vi "Sequence.BuildPreviewWaveform.vi"(7 "WaveformGraph in":refnum<vi>, 8 "error in (no error)":errorcluster, 9 "Rows":cluster{"Start Index":i32, "Length":i32}={"Start Index"=0, "Length"=-1}, 10 "UI.Sequence#ofColumns":i32, 11 "SequenceRef":refnum<vi>) -> (0 "error out":errorcluster, 2 "Wavefrom":waveform(dbl)[](array[waveform]))   [LabVIEW 2013, in "Simple Sequence Tools - Shared.lvlib"]
uses:
  Simple Sequence Tools - Shared.lvlib
  Main.Constants.vi
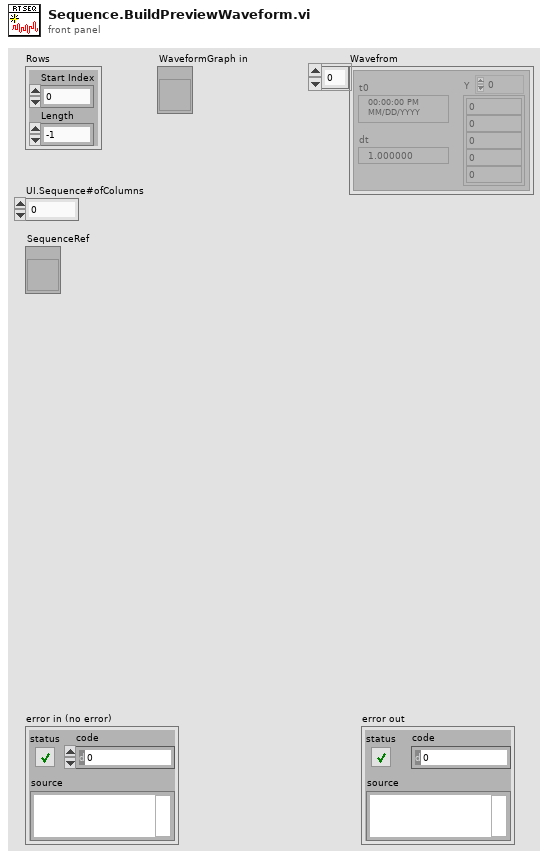
[diagram p1: front panel]
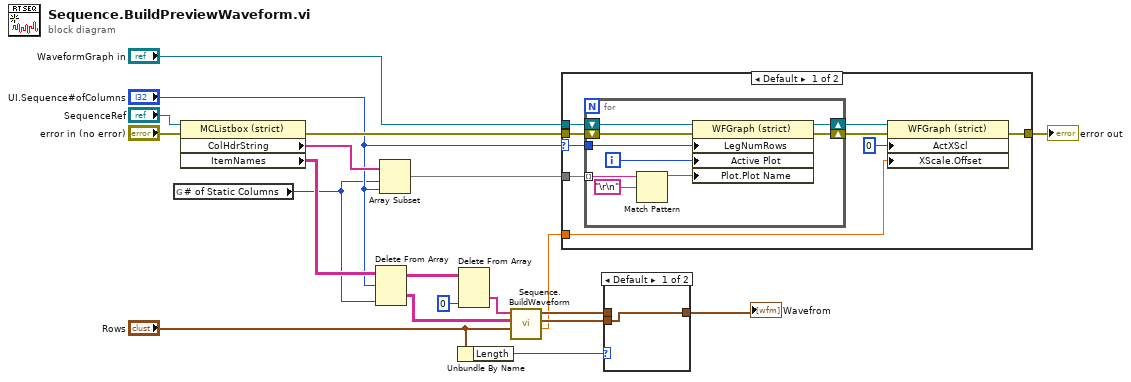
[diagram p0: block diagram]
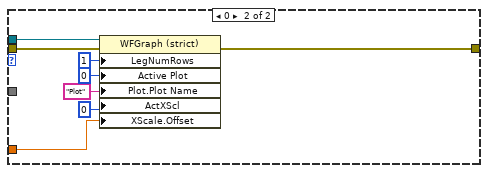
[diagram p3: hidden frame]
diagram:
  n1 = global read "Main.Constants.vi" "# of Static Columns"() -> (w1:u32)
  n2 = property class="MCListbox (strict)"(reference="SequenceRef", error in="error in (no error)") -> (error out=w12:errorcluster, "ColHdrString"=w14:string[], "ItemNames"=w11:string[][])  [unwired: 1 out]
  n3 = Delete From Array(array=w11, length="UI.Sequence#ofColumns", index (col)=w1) -> (deleted portion=w10:string[][], array with subset deleted=w17:string[][])  [unwired: 1 in]
  n4 = Array Subset(array=w14, index=w1, length="UI.Sequence#ofColumns") -> (w19:string[])
  n5 = Unbundle By Name("Rows") -> ("Length"=w5:i32)
  n6 = Delete From Array(array=w17, index (col)=0 ("disabled index (col)")) -> (deleted portion=w9:string[])  [unwired: 2 in, 1 out]
  n7 = call "Sequence.BuildWaveform.vi"("Rows"="Rows", "Steps"=w10, "Duration"=w9) -> ("Offset"=w2:dbl, "Selected"=w3:waveform(dbl)[], "Full"=w18:waveform(dbl)[])  [unwired: 6 in]
  n8 = case shown="Default" "UI.Sequence#ofColumns" {
    selector: "UI.Sequence#ofColumns" -> [w26 _]
    tunnel: [w24 w46] -> w20
    tunnel: w19 -> [w29 _]
    tunnel: "WaveformGraph in" -> [w28 w45]
    tunnel: w12 -> [w27 w44]
    tunnel: w2 -> [w21 w40]
    frame Default {
      n9 = for {
        tunnel: w26 -> [w38]
        tunnel: w29 -> [w35] mode=indexing
        shift-right: [w32] -> w25
        shift-left: w27 -> [w33]
        shift-right: [w30] -> w23
        shift-left: w28 -> [w31]
        i -> [w37]
        n10 = Match Pattern(string=w35, regular expression="\r\n") -> (before substring=w36:string)  [unwired: 1 in, 3 out]
        n11 = property on="Property Node" class="WFGraph (strict)"(reference=w31, error in=w33, "LegNumRows"=w38, "Active Plot"=w37, "Plot.Plot Name"=w36) -> (reference out=w30:refnum<vi>, error out=w32:errorcluster)
      }
      n12 = property on="Property Node" class="WFGraph (strict)"(reference=w23, error in=w25, "ActXScl"=0 ("Active X Scale"), "XScale.Offset"=w21) -> (error out=w24:errorcluster)  [unwired: 1 out]
    }
    frame 0 {
      n13 = property on="Property Node" class="WFGraph (strict)"(reference=w45, error in=w44, "LegNumRows"=u32 1 ("Legend:Number of Rows"), "Active Plot"=u32 0, "Plot.Plot Name"="Plot", "ActXScl"=0 ("Active X Scale"), "XScale.Offset"=w40) -> (error out=w46:errorcluster)  [unwired: 1 out]
    }
  }
  "error out" <- w20
  n14 = case shown="Default" w5 {
    tunnel: w18 -> [_ w48]
    tunnel: [w47 w48] -> w4
    tunnel: w3 -> [w47 _]
    frame Default {
    }
    frame -1 {
    }
  }
  "Wavefrom" <- w4
